vi "Global Stop.vi"() -> ()   [LabVIEW 2020]
panel:
  out "Global Stop":bool
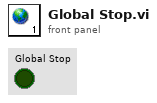
[diagram p1: front panel]
diagram:
